vi "UI Queue - Dequeue.vi"(8 "error in":errorcluster) -> (0 "error out":errorcluster, 1 "Message Data":variant, 2 "Message":string)   [LabVIEW 2024, in "User Interface.lvlib"]
uses:
  User Interface.lvlib
  Support/General Type Defs/FGV States.ctl
  Support/General Type Defs/General Type Defs.lvlib
  Support/QMH Messaging/QMH Messaging.lvlib
  Support/QMH Messaging/QMH - Dequeue Element.vi
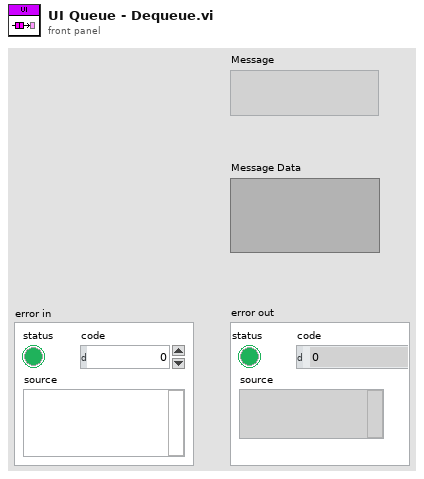
[diagram p1: front panel]
types:
  T1 = typedef "General Type Defs.lvlib/FGV States.ctl" = enum16{"Create", "Get", "Destroy"}
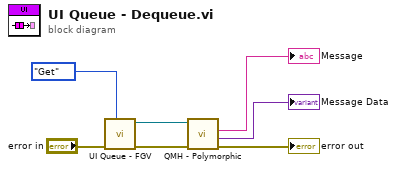
[diagram p0: block diagram]
diagram:
  n1 = call "UI Queue - FGV.vi"("FGV States"=FGV_States."Get", "error in"="error in") -> ("error out"=w7:errorcluster, "queue out"=w1:refnum<queue>)  [unwired: 8 in]
  n2 = call-poly "QMH - Polymorphic.vi"("error in (no error)"=w7, "Message Queue"=w1) -> ("error out"=→"error out":errorcluster, "Message Data"=→"Message Data":variant, "Message"=→"Message":string)  [unwired: 6 in, 1 out]
